vi "Read_image_and_encode_base64.vi"(11 "File Path":path) -> (3 "Base64 String":string)   [LabVIEW 2018]
panel:
  out "data":string
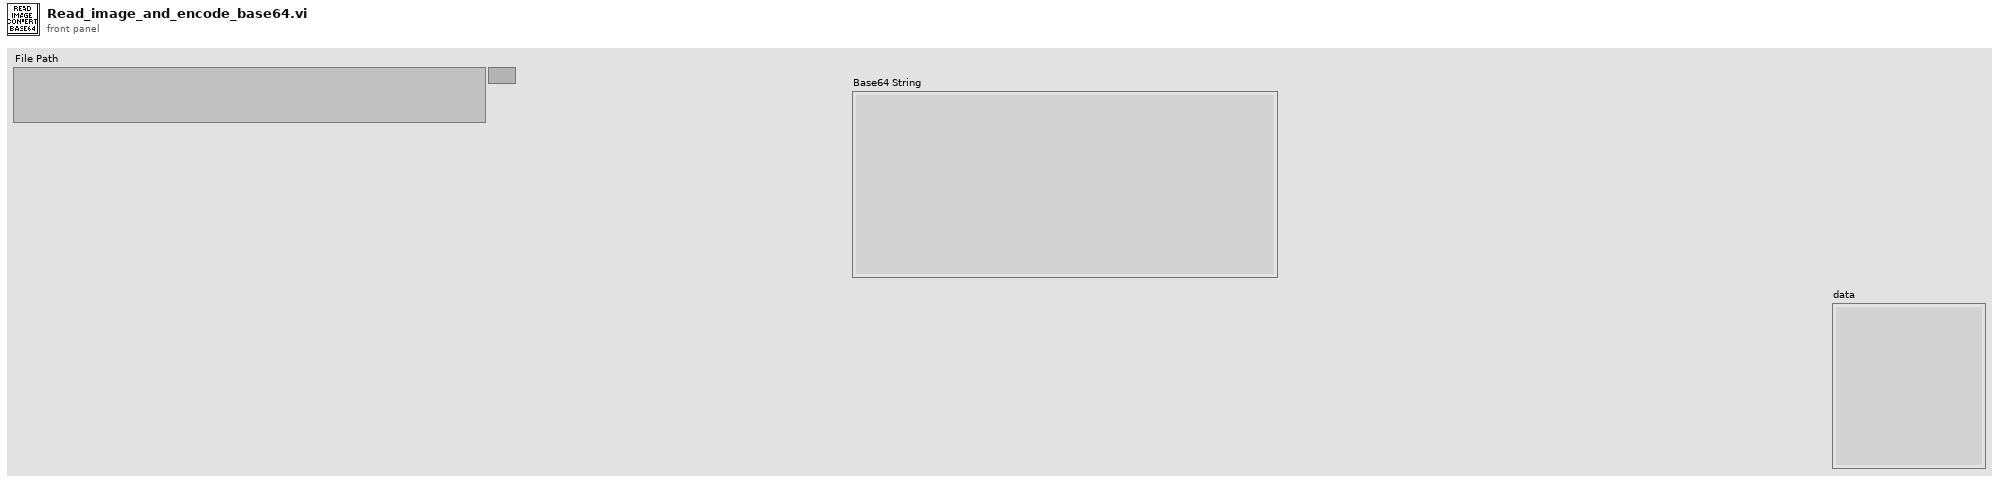
[diagram p1: front panel]
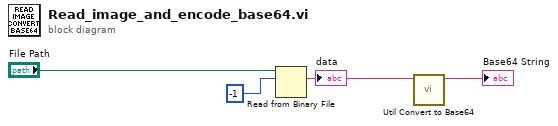
[diagram p0: block diagram]
diagram:
  n1 = Read from Binary File(10:-1 ("count (1)"), 11:"File Path") -> (2:w2:string)  [unwired: 4 in, 3 out]
  "data" <- w2
  n2 = call "Util Convert to Base64.vi"("String"=w2) -> ("Base64 String"=→"Base64 String":string)  [unwired: 10 in]
